vi "Error Query (Multiple).vi"(0 "VISA resource name":refnum<visa-resource-name>, 5 "error in (no error)":errorcluster) -> (14 "VISA resource name out":refnum<visa-resource-name>, 17 "Error":i32[](array[numeric]), 18 "Error Message":string, 19 "error out":errorcluster)   [LabVIEW 2020, in "Keithley 2100 Series.lvlib"]
doc: "This VI reads the error queue from the instrument. It expects to see errors in SCPI format (#,\"error message\"). It continues to read from the error queue until it reads a 0, \"No error\". If the instrument does not support an error query, a warning is returned."
uses:
  Keithley 2100 Series.lvlib
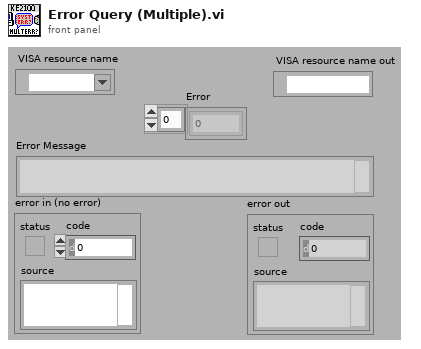
[diagram p1: front panel]
types:
  T1 = cluster{"Status":bool, "Error":i32, "source":string}
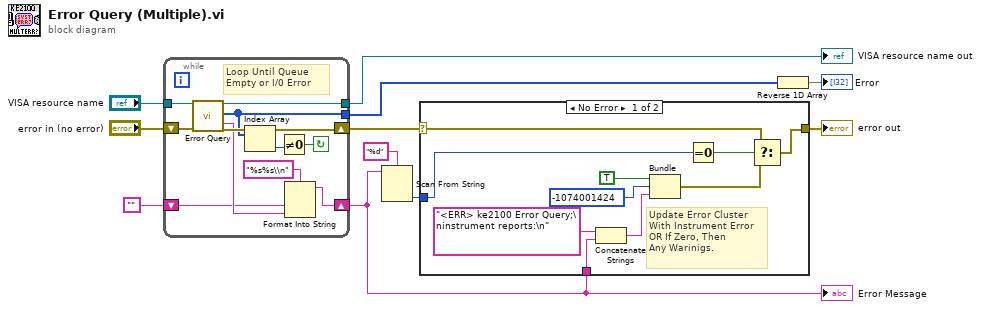
[diagram p0: block diagram]
diagram:
  n1 = while {
    tunnel: [w12] -> w9
    shift-left: "" ("Empty String Constant") -> [w16]
    shift-right: [w14] -> w3
    tunnel: "VISA resource name" -> [w20]
    tunnel: [w22] -> w7
    shift-right: [w18] -> w5
    shift-left: "error in (no error)" -> [w19]
    stop <- w21 continue-if-true
    # "Loop Until Queue Empty or I/0 Error"
    n2 = call "Error Query.vi"("VISA resource name"=w20, "error in (no error)"=w19) -> ("VISA resource name out"=w22:refnum<visa-resource-name>, "Error Code"=w12:i32[], "Error Message"=w17:string, "error out"=w18:errorcluster)  [unwired: 14 in]
    n3 = Index Array(array=w12) -> (element=w13:i32)  [unwired: 1 in]
    n4 = Not Equal To 0?(x=w13) -> (x != 0?=w21:bool)
    n5 = Format Into String(format string="%s%s\\n", w16, w17) -> (resulting string=w14:string)  [unwired: 2 in, 1 out]
  }
  "Error Message" <- w3
  "VISA resource name out" <- w7
  n6 = Scan From String(format string="%d", input string=w3) -> (output 1=w1:i32)  [unwired: 3 in, 3 out]
  n7 = case shown="No Error" w5 {
    selector: w5 -> [w23 w33]
    tunnel: w1 -> [w24 _]
    tunnel: [w26 w33] -> w10
    tunnel: w3 -> [w32 _]
    frame No Error {
      # "Update Error Cluster\nWith Instrument Error \nOR If Zero, Then \nAny Warinigs."
      n8 = Concatenate Strings("<ERR> ke2100 Error Query;\ninstrument reports:\n" ("Source"), w32) -> (w29:string)
      n9 = Bundle("Status"=TRUE, "Error"=-1074001424, w29) -> (w25:cluster{"Status":bool, "Error":i32, string})  [unwired: 1 in]
      n10 = Equal To 0?(x=w24) -> (x = 0?=w27:bool)
      n11 = Select(t=w23, s=w27, f=w25) -> (s? t:f=w26:T1)
    }
    frame Error {
      # "IO Error"
    }
  }
  "error out" <- w10
  n12 = Reverse 1D Array(array=w9) -> (reversed array=→"Error":i32[])
